vi "DrawSwitchesDELETEME.vi"(8 "error in (no error)":errorcluster, 11 "SnakeGame in":refnum<class "SnakeGame.lvclass">) -> (0 "error out":errorcluster, 3 "SnakeGame out":refnum<class "SnakeGame.lvclass">)   [LabVIEW 2019, in "RT_Game.lvlib" / "SnakeGame.lvclass"]
uses:
  SnakeGame.lvclass
  C:/Users/FreshBob/Dropbox/VIs/myRIO_GameConsole/RT/RT_Game/Game/Game.lvclass
  SnakeGame.lvclass/SnakeGame.ctl
  Snake/Snake.lvclass/Snake.ctl
  GameObject/GameObject.lvclass/GameObject.ctl
  PongSwitch/SnakeSwitch.lvclass/SnakeSwitch.ctl
  GameObject/Read position.vi
  PongSwitch/Write Tilecode.vi
  GameObject/Write IsActive.vi
  GameObject/Read name.vi
  GameObject/Read IsActive.vi
  PongSwitch/Read Toggled.vi
  PongSwitch/Read Tilecode.vi
  Snake/Read Position (Tiles).vi
  PongSwitch/SnakeSwitch.lvclass
  C:/Users/FreshBob/Dropbox/VIs/myRIO_GameConsole/RT/RT_Game/GameObject/GameObject.lvclass
  Game/Game.lvclass
  Snake/Snake.lvclass
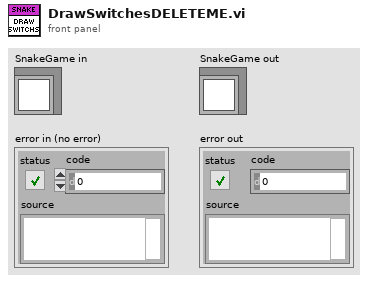
[diagram p1: front panel]
types:
  T1 = typedef "RT_Game.lvlib/Game.lvclass/Coordinate.ctl" = cluster{"x":dbl, "y":dbl}
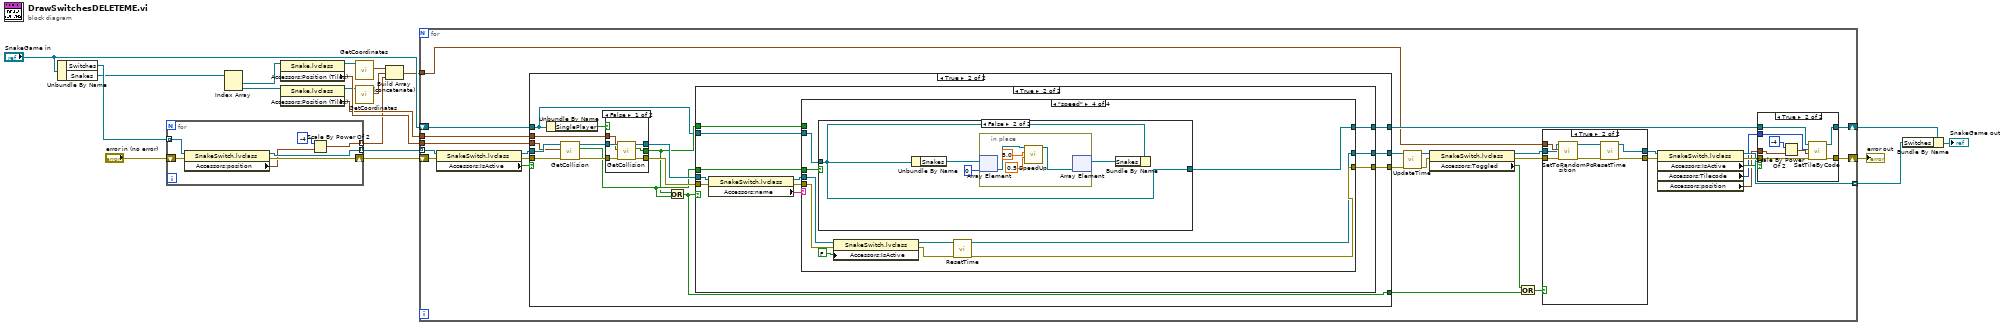
[diagram p0: block diagram]
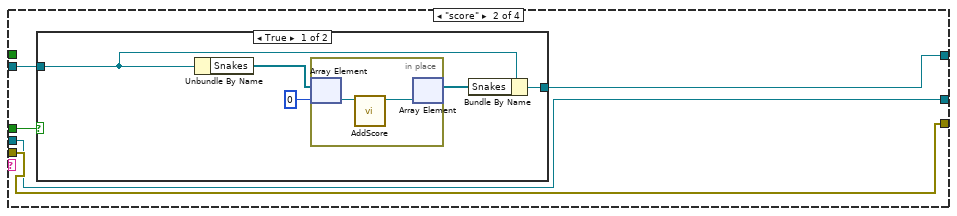
[diagram p7: hidden frame]
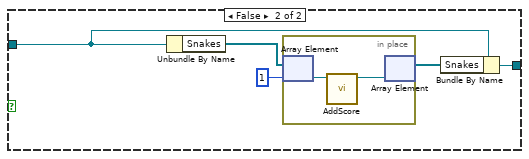
[diagram p8: hidden frame]
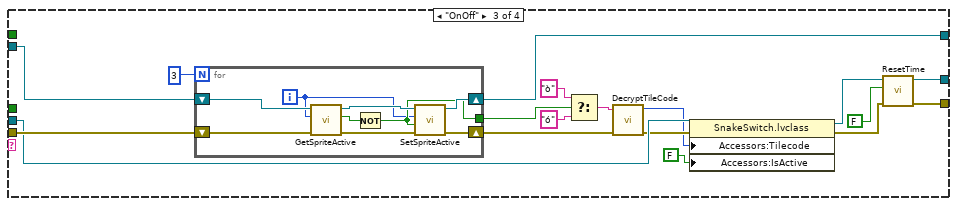
[diagram p9: hidden frame]
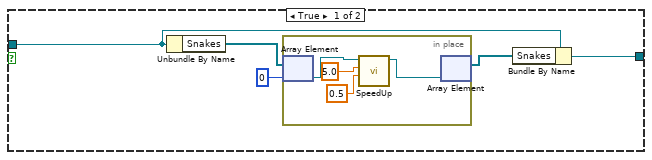
[diagram p10: hidden frame]
diagram:
  n1 = Unbundle By Name("SnakeGame in") -> ("Switches"=w20:refnum<class "SnakeSwitch.lvclass">[], "Snakes"=w5:refnum<class "Snake.lvclass">[])
  n2 = for {
    tunnel: [w25] -> w9 mode=indexing
    tunnel: w20 -> [w24] mode=indexing
    shift-right: [w26] -> w10
    shift-left: "error in (no error)" -> [w27]
    tunnel: [w22] -> w12 mode=indexing
    n3 = property class="SnakeSwitch.lvclass"(reference=w24, error in=w27) -> (reference out=w25:refnum<class "SnakeSwitch.lvclass">, error out=w26:errorcluster, "Accessors:position"=w23:T1)
    n4 = Scale By Power Of 2(n=i16 -4, x=w23) -> (x*2^n=w22:T1)
  }
  n5 = Index Array(array=w5) -> (element #1=w4:refnum<class "Snake.lvclass">, element #2=w3:refnum<class "Snake.lvclass">)  [unwired: 2 in]
  n6 = property class="Snake.lvclass"(reference=w4) -> (reference out=w2:refnum<class "Snake.lvclass">, "Accessors:Position (Tiles)"=w17:T1)  [unwired: 1 in, 1 out]
  n7 = property class="Snake.lvclass"(reference=w3) -> (reference out=w1:refnum<class "Snake.lvclass">, "Accessors:Position (Tiles)"=w16:T1)  [unwired: 1 in, 1 out]
  n8 = call "GetCoordinates.vi"("Snake in"=w2) -> ("Coordinates"=w7:T1[])  [unwired: 8 in, 2 out]
  n9 = call "GetCoordinates.vi"("Snake in"=w1) -> ("Coordinates"=w6:T1[])  [unwired: 8 in, 2 out]
  n10 = Build Array (concatenate)(w7, w6, w12) -> (w8:T1[])
  n11 = for {
    shift-right: [w55] -> w15
    shift-left: w10 -> [w28]
    shift-right: [w54] -> w14
    shift-left: "SnakeGame in" -> [w50]
    tunnel: w9 -> [w29] mode=indexing
    tunnel: w17 -> [w53]
    tunnel: w16 -> [w52]
    tunnel: w8 -> [w44]
    tunnel: [w35] -> w13 mode=indexing
    n12 = property class="SnakeSwitch.lvclass"(reference=w29, error in=w28) -> (reference out=w47:refnum<class "SnakeSwitch.lvclass">, error out=w48:errorcluster, "Accessors:IsActive"=w46:bool)
    n13 = case shown="True" w46 {
      tunnel: w48 -> [w66 w83]
      tunnel: w47 -> [w67 w82]
      tunnel: w53 -> [_ w78]
      tunnel: w52 -> [_ w77]
      tunnel: [w66 w76] -> w32
      tunnel: [w67 w74] -> w33
      tunnel: [w65 w73] -> w51
      tunnel: w50 -> [w65 w69]
      tunnel: [_ w68] -> w38
      frame False {
      }
      frame True {
        n14 = Unbundle By Name(w69) -> ("SinglePlayer"=w70:bool)
        n15 = call "GetCollision"("error in (no error)"=w83, "TilePosition"=w78, "PongSwitch in"=w82) -> ("error out"=w80:errorcluster, "Collided?"=w72:bool, "PongSwitch out"=w81:refnum<class "SnakeSwitch.lvclass">)  [unwired: 6 in]
        n16 = case shown="False" w70 {
          tunnel: w81 -> [w89 w91]
          tunnel: w80 -> [w88 w90]
          tunnel: [w87 w90] -> w79
          tunnel: w77 -> [w86 _]
          tunnel: [w85 w91] -> w75
          tunnel: [w84 _] -> w71
          frame False {
            n17 = call "GetCollision"("error in (no error)"=w88, "TilePosition"=w86, "PongSwitch in"=w89) -> ("error out"=w87:errorcluster, "Collided?"=w84:bool, "PongSwitch out"=w85:refnum<class "SnakeSwitch.lvclass">)  [unwired: 6 in]
          }
          frame True {
          }
        }
        n18 = Or(x=w71, y=w72) -> (x .or. y?=w68:bool)
        n19 = case shown="True" w68 {
          tunnel: w79 -> [w93 w95]
          tunnel: [w93 w105] -> w76
          tunnel: w75 -> [w94 w96]
          tunnel: [w94 w97] -> w74
          tunnel: [w92 w103] -> w73
          tunnel: w69 -> [w92 w104]
          tunnel: w72 -> [_ w100]
          tunnel: w71 -> [_ w99]
          frame False {
          }
          frame True {
            n20 = property class="SnakeSwitch.lvclass"(reference=w96, error in=w95) -> (reference out=w98:refnum<class "SnakeSwitch.lvclass">, error out=w102:errorcluster, "Accessors:name"=w101:string)
            n21 = case shown="\"speed\"" w101 {
              tunnel: w102 -> [w107 w113 w145 w164]
              tunnel: [w107 w113 w132 w161] -> w105
              tunnel: w104 -> [w108 w111 w143 w163]
              tunnel: [w108 w109 w133 w162] -> w103
              tunnel: w100 -> [_ w112 _ w155]
              tunnel: w99 -> [_ _ _ _]
              tunnel: w98 -> [w106 w110 w141 w158]
              tunnel: [w106 w110 w130 w160] -> w97
              frame Default {
              }
              frame "score" {
                n22 = case shown="True" w112 {
                  tunnel: w111 -> [w117 w124]
                  tunnel: [w118 w125] -> w109
                  frame True {
                    n23 = Unbundle By Name(w117) -> ("Snakes"=w116:refnum<class "Snake.lvclass">[])
                    n24 = in-place {
                      n25 = in-place-array #1(w116, 0) -> (w120:refnum<class "Snake.lvclass">)
                      n26 = call "AddScore.vi"("Snake in"=w120) -> ("Snake out"=w119:refnum<class "Snake.lvclass">)  [unwired: 9 in, 1 out]
                      n27 = in-place-array #1(w119) -> (w115:refnum<class "Snake.lvclass">[])  [unwired: 1 out]
                    }
                    n28 = Bundle By Name(cluster=w117, "Snakes"=w115) -> (w118:refnum<class "SnakeGame.lvclass">)
                  }
                  frame False {
                    n29 = Unbundle By Name(w124) -> ("Snakes"=w123:refnum<class "Snake.lvclass">[])
                    n30 = in-place {
                      n31 = in-place-array #2(w123, 1) -> (w127:refnum<class "Snake.lvclass">)
                      n32 = call "AddScore.vi"("Snake in"=w127) -> ("Snake out"=w126:refnum<class "Snake.lvclass">)  [unwired: 9 in, 1 out]
                      n33 = in-place-array #2(w126) -> (w122:refnum<class "Snake.lvclass">[])  [unwired: 1 out]
                    }
                    n34 = Bundle By Name(cluster=w124, "Snakes"=w122) -> (w125:refnum<class "SnakeGame.lvclass">)
                  }
                }
              }
              frame "OnOff" {
                n35 = for {
                  N: 3 -> [_]
                  tunnel: [w147] -> w136
                  shift-right: [w153] -> w144
                  shift-left: w145 -> [w154]
                  shift-right: [w152] -> w133
                  shift-left: w143 -> [w150]
                  i -> [w146]
                  n36 = call "GetSpriteActive.vi"("error in (no error)"=w154, "Index"=w146, "Game in"=w150) -> ("error out"=w151:errorcluster, "Active?"=w148:bool, "Game out"=w149:refnum<class "SnakeGame.lvclass">)  [unwired: 6 in]
                  n37 = Not(x=w148) -> (.not. x?=w147:bool)
                  n38 = call "SetSpriteActive.vi"("error in (no error)"=w151, "Active"=w147, "index"=w146, "Game in"=w149) -> ("error out"=w153:errorcluster, "Game out"=w152:refnum<class "SnakeGame.lvclass">)  [unwired: 6 in]
                }
                n39 = Select(t="ò" ("f"), s=w136, f="ó" ("TileCode")) -> (s? t:f=w139:string)
                n40 = call "DecryptTileCode.vi"("error in (no error)"=w144, "TileCode"=w139) -> ("error out"=w140:errorcluster, "TileCode"=w135:u16)  [unwired: 6 in, 2 out]
                n41 = property class="SnakeSwitch.lvclass"(reference=w141, error in=w140, "Accessors:Tilecode"=w135, "Accessors:IsActive"=FALSE ("IsActive")) -> (reference out=w131:refnum<class "SnakeSwitch.lvclass">, error out=w142:errorcluster)
                n42 = call "ResetTime.vi"("error in (no error)"=w142, "enabled"=FALSE, "SnakeSwitch in"=w131) -> ("error out"=w132:errorcluster, "SnakeSwitch out"=w130:refnum<class "SnakeSwitch.lvclass">)  [unwired: 7 in]
              }
              frame "speed" {
                n43 = case shown="False" w155 {
                  tunnel: w163 -> [w169 w177]
                  tunnel: [w168 w177] -> w162
                  frame True {
                    n44 = Unbundle By Name(w169) -> ("Snakes"=w167:refnum<class "Snake.lvclass">[])
                    n45 = in-place {
                      n46 = in-place-array #3(w167, 0) -> (w173:refnum<class "Snake.lvclass">)
                      n47 = call "SpeedUp.vi"("speed multiplier"=0.5, "Duration"=5.0, "Snake in"=w173) -> ("Snake out"=w172:refnum<class "Snake.lvclass">)  [unwired: 7 in, 1 out]
                      n48 = in-place-array #3(w172) -> (w166:refnum<class "Snake.lvclass">[])  [unwired: 1 out]
                    }
                    n49 = Bundle By Name(cluster=w169, "Snakes"=w166) -> (w168:refnum<class "SnakeGame.lvclass">)
                  }
                  frame False {
                    n50 = Unbundle By Name(w177) -> ("Snakes"=w176:refnum<class "Snake.lvclass">[])
                    n51 = in-place {
                      n52 = in-place-array #4(w176, 0) -> (w181:refnum<class "Snake.lvclass">)
                      n53 = call "SpeedUp.vi"("speed multiplier"=0.5, "Duration"=5.0, "Snake in"=w181) -> ("Snake out"=w180:refnum<class "Snake.lvclass">)  [unwired: 7 in, 1 out]
                      n54 = in-place-array #4(w180) -> (w175:refnum<class "Snake.lvclass">[])  [unwired: 1 out]
                    }
                    n55 = Bundle By Name(cluster=w177, "Snakes"=w175) -> ()  [unwired: 1 out]
                  }
                }
                n56 = property class="SnakeSwitch.lvclass"(reference=w158, error in=w164, "Accessors:IsActive"=FALSE ("IsActive")) -> (reference out=w157:refnum<class "SnakeSwitch.lvclass">, error out=w159:errorcluster)
                n57 = call "ResetTime.vi"("error in (no error)"=w159, "SnakeSwitch in"=w157) -> ("error out"=w161:errorcluster, "SnakeSwitch out"=w160:refnum<class "SnakeSwitch.lvclass">)  [unwired: 8 in]
              }
            }
          }
        }
      }
    }
    n58 = call "UpdateTime.vi"("error in (no error)"=w32, "SnakeSwitch in"=w33) -> ("error out"=w49:errorcluster, "SnakeSwitch out"=w42:refnum<class "SnakeSwitch.lvclass">)  [unwired: 8 in]
    n59 = property class="SnakeSwitch.lvclass"(reference=w42, error in=w49) -> (reference out=w41:refnum<class "SnakeSwitch.lvclass">, error out=w43:errorcluster, "Accessors:Toggled"=w40:bool)
    n60 = Or(x=w40, y=w38) -> (x .or. y?=w39:bool)
    n61 = case shown="True" w39 {
      tunnel: [w56 w60] -> w45
      tunnel: [w57 w58] -> w36
      tunnel: w44 -> [_ w63]
      tunnel: w43 -> [w56 w62]
      tunnel: w41 -> [w57 w61]
      frame False {
      }
      frame True {
        n62 = call "SetToRandomPosition.vi"("error in (no error)"=w62, "BlockedSpots"=w63, "SnakeSwitch in"=w61) -> ("error out"=w64:errorcluster, "SnakeSwitch out"=w59:refnum<class "SnakeSwitch.lvclass">)  [unwired: 7 in]
        n63 = call "ResetTime.vi"("error in (no error)"=w64, "SnakeSwitch in"=w59) -> ("error out"=w60:errorcluster, "SnakeSwitch out"=w58:refnum<class "SnakeSwitch.lvclass">)  [unwired: 8 in]
      }
    }
    n64 = property class="SnakeSwitch.lvclass"(reference=w36, error in=w45) -> (reference out=w35:refnum<class "SnakeSwitch.lvclass">, error out=w37:errorcluster, "Accessors:IsActive"=w34:bool, "Accessors:Tilecode"=w31:u16, "Accessors:position"=w30:T1)
    n65 = case shown="True" w34 {
      tunnel: [w182 w191] -> w55
      tunnel: [w183 w190] -> w54
      tunnel: w37 -> [w182 w189]
      tunnel: w51 -> [w183 w188]
      tunnel: w30 -> [_ w187]
      tunnel: w31 -> [_ w184]
      frame False {
      }
      frame True {
        n66 = Scale By Power Of 2(n=i16 -4, x=w187) -> (x*2^n=w185:T1)
        n67 = call "SetTileByCode.vi"("error in (no error)"=w189, "Coordinates"=w185, "TileNumber"=w184, "Game in"=w188) -> ("error out"=w191:errorcluster, "Game out"=w190:refnum<class "SnakeGame.lvclass">)  [unwired: 6 in]
      }
    }
  }
  "error out" <- w15
  n68 = Bundle By Name(cluster=w14, "Switches"=w13) -> (→"SnakeGame out":refnum<class "SnakeGame.lvclass">)
